vi "Query Instrument Status.vi"(8 "error in (no error)":errorcluster, 11 "VISA resource name":refnum<visa-resource-name>) -> (0 "error out":errorcluster, 2 "Questionable Data Message":string, 3 "VISA resource name out":refnum<visa-resource-name>)   [LabVIEW 2013, in "DmmPwr Simulator.lvlib"]
doc: "Gets the instrument status from the instrument."
uses:
  <instrlib>/DmmPwr Simulator/DmmPwr Simulator.lvlib
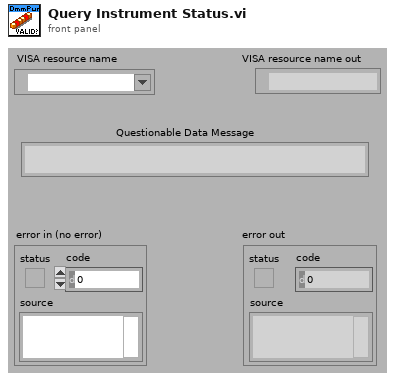
[diagram p1: front panel]
types:
  T1 = cluster{"Boolean array[0]":bool, "Boolean array[1]":bool, "Boolean array[2]":bool, "Boolean array[3]":bool, "Boolean array[4]":bool, "Boolean array[5]":bool, "Boolean array[6]":bool, "Boolean array[7]":bool, "Boolean array[8]":bool, "Boolean array[9]":bool, "Boolean array[10]":bool, "Boolean array[11]":bool, "Boolean array[12]":bool, "Boolean array[13]":bool, "Boolean array[14]":bool, "Boolean array[15]":bool}
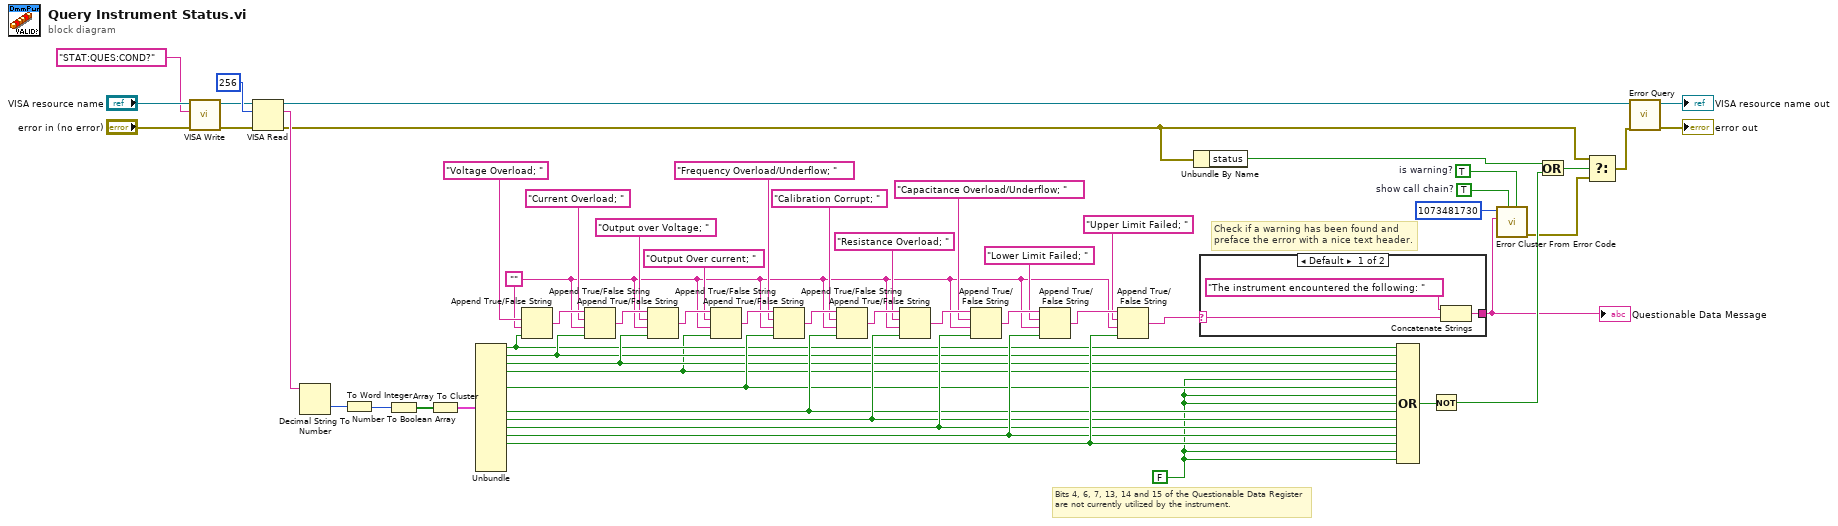
[diagram p0: block diagram]
diagram:
  w20 = TRUE  # is warning?
  w21 = TRUE  # show call chain?
  w16 = FALSE
  w34 = ""
  # "Check if a warning has been found and preface the error with a nice text header."
  # "Bits 4, 6, 7, 13, 14 and 15 of the Questionable Data Register are not currently utilized by the instrument."
  n1 = call <instrlib>:"VISA Write.vi"("error in"="error in (no error)", "write buffer"="STAT:QUES:COND?", "VISA resource name"="VISA resource name") -> ("error out"=w5:errorcluster, "VISA resource name out"=w6:refnum<visa-resource-name>)  [unwired: 6 in, 1 out]
  n2 = VISA Read(VISA resource name=w6, byte count=u32 256, error in (no error)=w5) -> (VISA resource name out=w4:refnum<visa-resource-name>, read buffer=w18:string, error out=w11:errorcluster)  [unwired: 1 out]
  n3 = Decimal String To Number(string=w18) -> (number=w55:i32)  [unwired: 3 out]
  n4 = To Word Integer(number=w55) -> (16bit integer=w56:i16)
  n5 = Number To Boolean Array(number=w56) -> (Boolean array=w57:bool[])
  n6 = Array To Cluster(array=w57) -> (cluster=w54:T1)
  n7 = Unbundle(w54) -> ("Boolean array[0]"=w25:bool, "Boolean array[1]"=w26:bool, "Boolean array[2]"=w27:bool, "Boolean array[3]"=w17:bool, "Boolean array[5]"=w28:bool, "Boolean array[8]"=w29:bool, "Boolean array[9]"=w30:bool, "Boolean array[10]"=w31:bool, "Boolean array[11]"=w32:bool, "Boolean array[12]"=w33:bool)  [unwired: 6 out]
  n8 = Append True/False String(1:w25, 2:w34, 3:"Voltage Overload; " ("true string")) -> (0:w53:string)  [unwired: 1 out]
  n9 = Append True/False String(1:w26, 2:w34, 3:"Current Overload; " ("true string"), 4:w53) -> (0:w52:string)
  n10 = Append True/False String(1:w27, 2:w34, 3:"Output over Voltage; " ("true string"), 4:w52) -> (0:w51:string)
  n11 = Append True/False String(1:w17, 2:w34, 3:"Output Over current; " ("true string"), 4:w51) -> (0:w50:string)
  n12 = Append True/False String(1:w28, 2:w34, 3:"Frequency Overload/Underflow; " ("true string"), 4:w50) -> (0:w49:string)
  n13 = Append True/False String(1:w29, 2:w34, 3:"Calibration Corrupt; " ("true string"), 4:w49) -> (0:w48:string)
  n14 = Append True/False String(1:w30, 2:w34, 3:"Resistance Overload; " ("true string"), 4:w48) -> (0:w47:string)
  n15 = Append True/False String(1:w31, 2:w34, 3:"Capacitance Overload/Underflow; " ("true string"), 4:w47) -> (0:w46:string)
  n16 = Append True/False String(1:w32, 2:w34, 3:"Lower Limit Failed; " ("true string"), 4:w46) -> (0:w45:string)
  n17 = Append True/False String(1:w33, 2:w34, 3:"Upper Limit Failed; " ("true string"), 4:w45) -> (0:w15:string)
  n18 = Unbundle By Name(w11) -> ("status"=w13:bool)
  n19 = case shown="Default" w15 {
    selector: w15 -> [w59 w61]
    tunnel: [w58 w61] -> w14
    frame Default {
      n20 = Concatenate Strings("The instrument encountered the following: " ("true string"), w59) -> (w58:string)
    }
    frame "" {
    }
  }
  "Questionable Data Message" <- w14
  n21 = Compound Arithmetic op=OR(w25, w26, w27, w17, w16, w28, w16, w16, w29, w30, w31, w32, w33, w16, w16) -> (w24:bool)
  n22 = Not(x=w24) -> (.not. x?=w23:bool)
  n23 = call <vilib>:"Error Cluster From Error Code.vi"("is warning? (False)"=w20, "show call chain? (False)"=w21, "error message (\"\")"=w14, "error code (0)"=1073481730 ("t")) -> ("error out"=w10:errorcluster)  [unwired: 1 in, 4 out]
  n24 = Or(x=w13, y=w23) -> (x .or. y?=w12:bool)
  n25 = Select(t=w11, s=w12, f=w10) -> (s? t:f=w1:errorcluster)
  n26 = call <instrlib>:"Error Query.vi"("error in (no error)"=w1, "VISA resource name"=w4) -> ("error out"=→"error out":errorcluster, "VISA resource name out"=→"VISA resource name out":refnum<visa-resource-name>)  [unwired: 6 in, 2 out]
